vi "PH_ImageOperator.Subtract Background Image.vi"(0 "i ref in":refnum<vi>, 2 "Cam Image":T1, 5 "error in (no error)":errorcluster) -> (14 "i ref out":refnum<vi>, 19 "error out":errorcluster)   [LabVIEW 2014, in "PH_ImageOperator.lvlib"]
doc: "This VI subtracts the background image (if available). Together with the information whether this has been successful it saves the raw image and the final image to own attributes."
uses:
  PH_ImageOperator.lvlib
  <vilib>/vision/Image Controls.llb/IMAQ Image.ctl
  PH_StatusHandler/PH_StatusHandler.Status.ctl
  PH_Common/PH_Common.lvlib
  <vilib>/vision/NI_Vision_Development_Module.lvlib
  PH_StatusHandler/PH_StatusHandler.lvlib
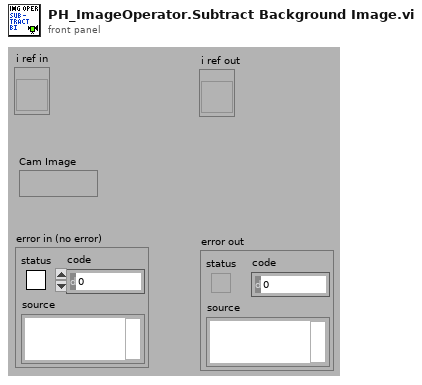
[diagram p1: front panel]
types:
  T1 = typedef "IMAQ Image.ctl" = refnum<image>
  T2 = typedef "PH_ImageOperator.lvlib/PH_ImageOperator.i attribute.ctl" = cluster{"GUI Refs":cluster{"Delete":refnum<vi>, "Calibration status":refnum<vi>, "BI subtracted":refnum<vi>, "calc Energy":refnum<vi>, "Energy: expected value":refnum<vi>, "Energy: Tolerance":refnum<vi>, "Energy calculated":refnum<vi>, "Energy":refnum<vi>, "calc Beam Anal":refnum<vi>, "Maj Diam 1/esquare":refnum<vi>, "Min Diam 1/esquare":refnum<vi>, "Azi Angle":refnum<vi>, "Min/Maj Diam esquare":refnum<vi>, "Beam analysed":refnum<vi>, "CoG - x":refnum<vi>, "CoG - y":refnum<vi>, "BA: Method":refnum<vi>, "BA: Steps":refnum<vi>, "BA: Factor":refnum<vi>, "calc Traces":refnum<vi>, "Traces: Fit Gauss":refnum<vi>, "Traces calculated":refnum<vi>, "Maj FWHM":refnum<vi>, "Min FWHM":refnum<vi>, "Major Trace":refnum<vi>, "Minor Trace":refnum<vi>, "Maj Fit Order":refnum<vi>, "Min Fit Order":refnum<vi>, "Position calculated":refnum<vi>, "Position":refnum<vi>, "Type":refnum<vi>, "Center":refnum<vi>, "exp - X":refnum<vi>, "exp - Y":refnum<vi>, "Tolerance":refnum<vi>, "f":refnum<vi>, "M":refnum<vi>, "D":refnum<vi>, "q":refnum<vi>, "Dummy Method":refnum<vi>, "Dummy Type":refnum<vi>, "Global On":refnum<vi>, "Traces: No offset":refnum<vi>, "Maj 99%":refnum<vi>, "Min 99%":refnum<vi>, "GUI FF Image":refnum<vi>, "calc Fill Factor":refnum<vi>, "FF calculated":refnum<vi>, "Fill Factor: Filter?":refnum<vi>, "FF: Damage Threshold":refnum<vi>, "FF: Threshold":refnum<vi>, "FF: max allow. Energy":refnum<vi>, "FF: Fillfactor":refnum<vi>, "Calibration data":refnum<vi>}, "List of GUIs":string[], "Calibration":cluster{"Status":T3, "Calibration data":T4, "Calibration Data File":path}, "Final Image":cluster{"BI Subtraction Failure":bool}, "Energy":cluster{"on":bool, "expected value [mJ]":dbl, "Tolerance [%]":dbl, "State":T3, "Energy [mJ]":dbl, "Unit":string, "calculated @":timestamp}, "Beam Analysis":cluster{"on":bool, "Data":T5, "Method":bool, "Steps":i32, "Factor":i32, "ROI":cluster{"Left":i32, "Top":i32, "Right":i32, "Bottom":i32}, "analysed @":timestamp}, "Trace Analysis":cluster{"on":bool, "Fit on":bool, "Maj FWHM":dbl, "Min FWHM":dbl, "Maj Fit Order":i32, "Min Fit Order":i32, "No Offset":bool, "Maj 99%":dbl, "Min 99%":dbl, "Traces":cluster{"XScaleName":string, "Y Scale Minimum":sgl, "Y Scale Maximum":sgl, "X Scale Minimum":sgl, "X Scale Maximum":sgl, "Traces":cluster{"Index":sgl[], "Trace":dbl[]}[]}[], "analysed @":timestamp}, "Position Analysis":cluster{"on":bool, "exp - X":i32, "exp - Y":i32, "focal length [mm]":dbl, "Magnification":dbl, "Delta":dbl, "Theta":dbl, "Tolerance":dbl, "Type":bool, "analysed @":timestamp}, "Fill Factor":cluster{"on":bool, "Filter on?":bool, "Threshold":dbl, "Damage Threshold [J/cm²]":dbl, "Fillfactor":dbl, "Max. allowed Energy [J]":dbl, "calculated @":timestamp}, "Statistician Service ID":i32, "Images":cluster{"Background":T1, "OP":T1, "GUI":T1, "BA: ROI":T1, "Trace: Turn":T1, "FF: Main":T1, "FF: Help":T1, "PSDB: BG":T1, "PSDB: OP":T1, "PSDB: FF":T1}}
  T3 = typedef "PH_StatusHandler.lvlib/PH_StatusHandler.Status.ctl" = i16
  T4 = typedef "PH_ImageCalibrator.lvlib/PH_ImageCalibrator.Calibration Data.ctl" = cluster{"Date":string, "Time":string, "Cam Settings":cluster{"Cam ID":string, "Gain":dbl, "Brightness":dbl, "Shutter":dbl, "Cam Error":bool, "Mode":i32}, "Background Image":cluster{"Image":dbl[][], "Image Error":bool}, "Linear Calibration":cluster{"Calibration Factor":dbl, "not mm or mrad":bool}, "Energy Calibration":cluster{"Calibration Factor":dbl, "no mJ":bool}}
  T5 = typedef "PH_ImageOperator.lvlib/PH_ImageOperator.Beam Analysis Data.ctl" = cluster{"CoG-x":sgl, "CoG-y":sgl, "Maj Dim":dbl, "Min Dim":dbl, "Ellipticity":dbl, "Azimuth Angle [rad]":dbl, "Azi Angle rel to Maj?":bool}
  T6 = typedef "Image Type" = u32
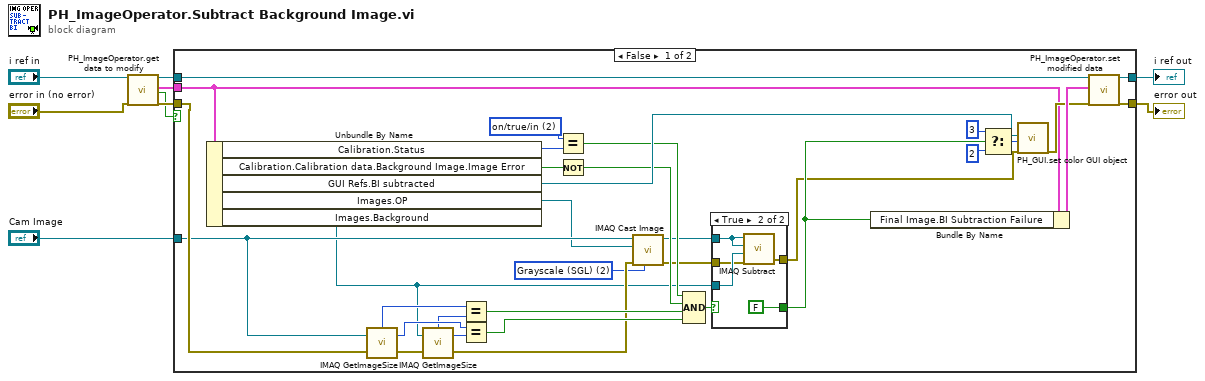
[diagram p0: block diagram]
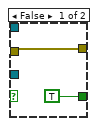
[diagram p2: hidden frame]
diagram:
  n1 = call "PH_ImageOperator.get data to modify.vi"("i ref in"="i ref in", "error in (no error)"="error in (no error)") -> ("i ref out"=w8:refnum<vi>, "i attribute"=w5:T2, "timed out"=w4:bool, "error out"=w9:errorcluster)  [unwired: 14 in]
  n2 = case shown="False" w4 {
    tunnel: w9 -> [w20 w50]
    tunnel: w8 -> [w42 w51]
    tunnel: [w41 w51] -> w7
    tunnel: [w40 w50] -> w6
    tunnel: w5 -> [w33 _]
    tunnel: "Cam Image" -> [w14 _]
    frame False {
      w12 = T6 2 items=["Grayscale (U8)", "Grayscale (I16)", "Grayscale (SGL)", "Complex (CSG)", "RGB (U32)", "HSL (U32)", "RGB (U64)"] ("Image Type")
      w22 = T3 2 items=["no info", "off/false/out", "on/true/in", "Failure", "Alarm", "Status 1", "Status 2", "Status 3"] ("Calibration.Status")
      n3 = Unbundle By Name(w33) -> ("Calibration.Status"=w23:T3, "Calibration.Calibration data.Background Image.Image Error"=w34:bool, "GUI Refs.BI subtracted"=w21:refnum<vi>, "Images.OP"=w11:T1, "Images.Background"=w10:T1)
      n4 = call "IMAQ GetImageSize"("Image"=w14, "error in (no error)"=w20) -> ("Y Resolution"=w28:i32, "X Resolution"=w26:i32, "error out"=w25:errorcluster)  [unwired: 2 in]
      n5 = call "IMAQ GetImageSize"("Image"=w10, "error in (no error)"=w25) -> ("Y Resolution"=w29:i32, "X Resolution"=w27:i32, "error out"=w16:errorcluster)  [unwired: 2 in]
      n6 = Equal?(x=w26, y=w27) -> (x = y?=w30:bool)
      n7 = Equal?(x=w28, y=w29) -> (x = y?=w31:bool)
      n8 = Equal?(x=w22, y=w23) -> (x = y?=w17:bool)
      n9 = Not(x=w34) -> (.not. x?=w18:bool)
      n10 = call "IMAQ Cast Image"("Image Type"=w12, "error in (no error)"=w16, "Image Dst"=w11, "Image Src"=w14) -> ("error out"=w15:errorcluster, "Image Dst Out"=w13:T1)  [unwired: 6 in]
      n11 = Compound Arithmetic op=AND(w17, w18, w30, w31) -> (w32:bool)
      n12 = case shown="True" w32 {
        tunnel: w10 -> [_ w48]
        tunnel: w13 -> [_ w47]
        tunnel: [TRUE FALSE] -> w24
        tunnel: w15 -> [w44 w46]
        tunnel: [w44 w49] -> w19
        frame False {
        }
        frame True {
          n13 = call "IMAQ Subtract"("Image Src A"=w47, "Image Dst"=w47, "Image Src B"=w48, "error in (no error)"=w46) -> ("error out"=w49:errorcluster)  [unwired: 3 in, 1 out]
        }
      }
      n14 = Bundle By Name(cluster=w33, "Final Image.BI Subtraction Failure"=w24) -> (w39:T2)
      n15 = Select(t=3, s=w24, f=2) -> (s? t:f=w37:i32)
      n16 = call "PH_GUI.set color GUI object.vi"("GUI object Ref"=w21, "State"=w37, "error in (no error)"=w19) -> ("error out"=w38:errorcluster)  [unwired: 16 in]
      n17 = call "PH_ImageOperator.set modified data.vi"("i ref in"=w42, "i attribute"=w39, "error in (no error)"=w38) -> ("i ref out"=w41:refnum<vi>, "error out"=w40:errorcluster)  [unwired: 15 in]
    }
    frame True {
    }
  }
  "error out" <- w6
  "i ref out" <- w7
